vi "Stop System.vi"(8 "error in (no error)":errorcluster) -> (0 "error out":errorcluster)   [LabVIEW 2016, in "System.lvlib"]
uses:
  System.lvlib
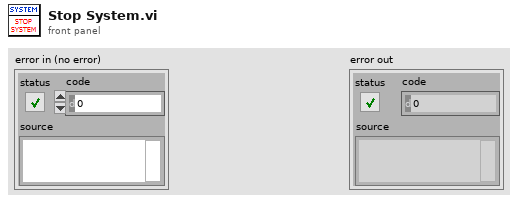
[diagram p1: front panel]
types:
  T1 = typedef "System.lvlib/Control_User Event.ctl" = cluster{"Stop":refnum<user-event>, "Error":refnum<user-event>}
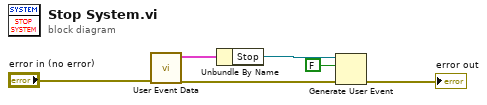
[diagram p0: block diagram]
diagram:
  n1 = call "User Event Data.vi"("error in (no error)"="error in (no error)") -> ("error out"=w4:errorcluster, "User Event Data"=w5:T1)  [unwired: 9 in]
  n2 = Unbundle By Name(w5) -> ("Stop"=w3:refnum<user-event>)
  n3 = Generate User Event(user event=w3, event data cluster=FALSE, error in=w4) -> (error out=→"error out":errorcluster)  [unwired: 1 in, 1 out]
